vi "Deserialize Core.vi"(8 "error in (no error)":errorcluster, 10 "Serialized Attributes":string, 11 "Serialize in":refnum<class "echo Msg.lvclass">) -> (0 "error out":errorcluster, 3 "Serialize out":refnum<class "echo Msg.lvclass">)   [LabVIEW 2020, in "Chat Window.lvlib" / "echo Msg.lvclass"]
uses:
  echo Msg.lvclass
  echo Msg.lvclass/echo Msg.ctl
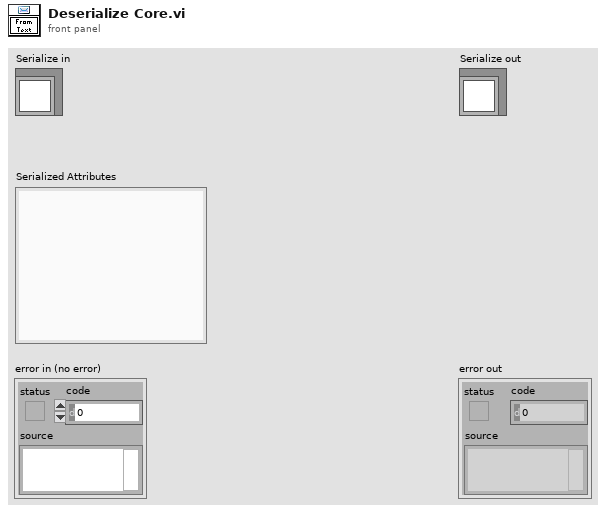
[diagram p1: front panel]
types:
  T1 = cluster{"Message":string, "id":string, "exec_time":i32}
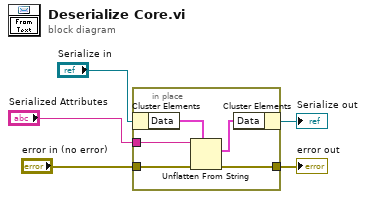
[diagram p0: block diagram]
diagram:
  n1 = in-place "In Place Element Structure" {
    in-place-border: "Serialized Attributes" -> [w7]
    in-place-border: "error in (no error)" -> [w10]
    in-place-border: [w9] -> w1
    n2 = in-place-cluster #1("Serialize in") -> ("Data"=w8:T1)
    n3 = Unflatten From String(type=w8, binary string=w7, error in (no error)=w10) -> (value=w6:T1, error out=w9:errorcluster)  [unwired: 2 in, 1 out]
    n4 = in-place-cluster #1("Data"=w6) -> (→"Serialize out":refnum<class "echo Msg.lvclass">)
  }
  "error out" <- w1
